vi "Add Log.vi"(6 "Time (Now)":dbl, 8 "error in (no error)":errorcluster, 9 "Message":string, 10 "From (Client)":string, 11 "LV Chat Client in":refnum<class "LV Chat Client.lvclass">) -> (0 "error out":errorcluster, 3 "LV Chat Client out":refnum<class "LV Chat Client.lvclass">)   [LabVIEW 2020, in "LV Chat Client.lvclass"]
uses:
  LV Chat Client.lvclass
  Data Types/Message.ctl
  LV Chat Client.lvclass/LV Chat Client.ctl
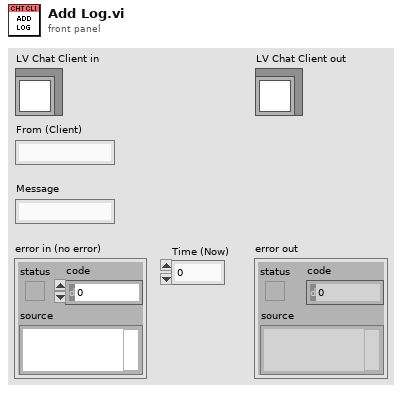
[diagram p1: front panel]
types:
  T1 = typedef "Message.ctl" = cluster{"From":string, "Time":dbl, "Message":string}
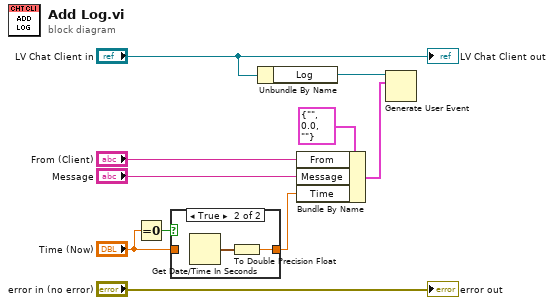
[diagram p0: block diagram]
diagram:
  n1 = Equal To 0?(x="Time (Now)") -> (x = 0?=w9:bool)
  n2 = case shown="True" w9 {
    tunnel: "Time (Now)" -> [w11 _]
    tunnel: [w11 w12] -> w4
    frame False {
    }
    frame True {
      n3 = Get Date/Time In Seconds() -> (seconds since 1Jan1904=w13:timestamp)
      n4 = To Double Precision Float(number=w13) -> (double precision float=w12:dbl)
    }
  }
  n5 = Unbundle By Name("LV Chat Client in") -> ("Log"=w2:refnum<user-event>)
  n6 = Bundle By Name(cluster=T1 {"From"="", "Time"=0.0, "Message"=""} ("Message"), "From"="From (Client)", "Message"="Message", "Time"=w4) -> (w1:T1)
  n7 = Generate User Event(user event=w2, event data cluster=w1) -> ()  [unwired: 2 in, 2 out]
  "error out" <- "error in (no error)"
  "LV Chat Client out" <- "LV Chat Client in"
